vi "updatestats.vi"(8 "error in (no error)":errorcluster, 10 "Stats Ref":refnum<vi>, 11 "Result Ref":refnum<vi>) -> (0 "error IO":errorcluster, 3 "result ref out":refnum<vi>)   [LabVIEW 2022 SP3]
uses:
  <vilib>/Analysis/NI_AALBase.lvlib
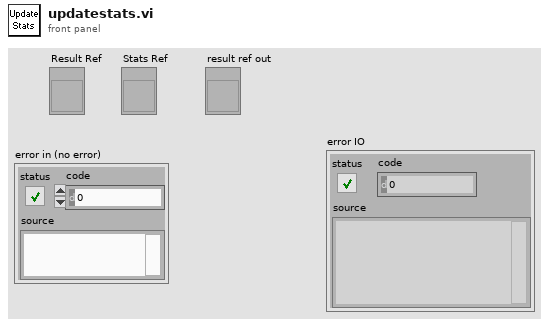
[diagram p1: front panel]
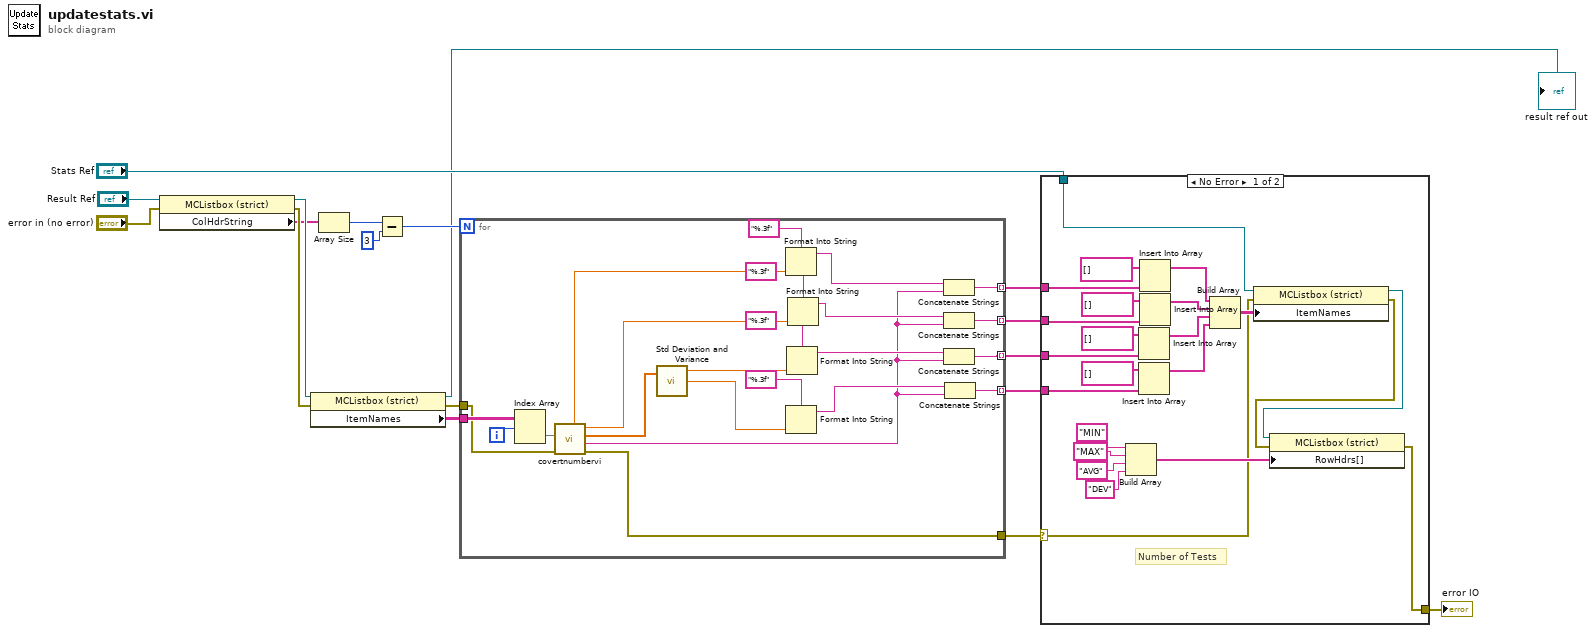
[diagram p0: block diagram]
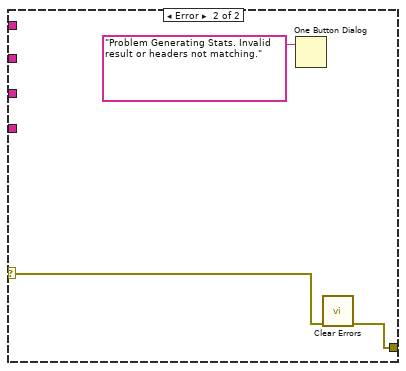
[diagram p2: hidden frame]
diagram:
  n1 = property class="MCListbox (strict)"(reference="Result Ref", error in="error in (no error)") -> (reference out=w15:refnum<vi>, error out=w18:errorcluster, "ColHdrString"=w14:string[])
  n2 = property class="MCListbox (strict)"(reference=w15, error in=w18) -> (reference out=→"result ref out":refnum<vi>, error out=w17:errorcluster, "ItemNames"=w16:string[][])
  n3 = Array Size(array=w14) -> (size(s)=w10:i32)
  n4 = Subtract(x=w10, y=u32 3) -> (x-y=w7:u32)
  n5 = for {
    N: w7 -> [_]
    tunnel: w16 -> [w41]
    tunnel: w17 -> [w28]
    tunnel: [w29] -> w13
    tunnel: [w32] -> w8 mode=indexing
    tunnel: [w31] -> w9 mode=indexing
    tunnel: [w37] -> w11 mode=indexing
    tunnel: [w34] -> w12 mode=indexing
    i -> [w40]
    n6 = Index Array(array=w41, index (col)=w40) -> (element=w27:string[])  [unwired: 1 in]
    n7 = call "covertnumbervi.vi"("error in"=w28, "Array"=w27) -> ("error out"=w29:errorcluster, "Symbol"=w26:string, "Array Out"=w23:dbl[], "max value"=w24:dbl, "min value"=w25:dbl)  [unwired: 4 in]
    n8 = call <vilib>:"Std Deviation and Variance.vi"("X"=w23) -> ("mean"=w38:dbl, "standard deviation"=w36:dbl)  [unwired: 1 in, 1 out]
    n9 = Format Into String(format string="%.3f", w25) -> (resulting string=w33:string)  [unwired: 2 in, 1 out]
    n10 = Format Into String(format string="%.3f", w36) -> (resulting string=w35:string)  [unwired: 2 in, 1 out]
    n11 = Format Into String(format string="%.3f", w38) -> (resulting string=w39:string)  [unwired: 2 in, 1 out]
    n12 = Format Into String(format string="%.3f", w24) -> (resulting string=w30:string)  [unwired: 2 in, 1 out]
    n13 = Concatenate Strings(w33, w26) -> (w32:string)
    n14 = Concatenate Strings(w30, w26) -> (w31:string)
    n15 = Concatenate Strings(w39, w26) -> (w37:string)
    n16 = Concatenate Strings(w35, w26) -> (w34:string)
  }
  n17 = case shown="No Error" w13 {
    selector: w13 -> [w45 w66]
    tunnel: [w47 w65] -> w2
    tunnel: w8 -> [w58 _]
    tunnel: w9 -> [w57 _]
    tunnel: w11 -> [w54 _]
    tunnel: w12 -> [w52 _]
    tunnel: "Stats Ref" -> [w50 _]
    frame No Error {
      # "Number of Tests"
      n18 = Build Array("MIN", "MAX", "AVG", "DEV") -> (w48:string[])
      n19 = Insert Into Array(array=string[] [], new element=w54) -> (w55:string[])  [unwired: 1 in]
      n20 = Insert Into Array(array=string[] [], new element=w52) -> (w51:string[])  [unwired: 1 in]
      n21 = Insert Into Array(array=string[] [], new element=w58) -> (w43:string[])  [unwired: 1 in]
      n22 = Insert Into Array(array=string[] [], new element=w57) -> (w42:string[])  [unwired: 1 in]
      n23 = Build Array(w43, w42, w55, w51) -> (w49:string[][])
      n24 = property class="MCListbox (strict)"(reference=w50, error in=w45, "ItemNames"=w49) -> (reference out=w44:refnum<vi>, error out=w46:errorcluster)
      n25 = property class="MCListbox (strict)"(reference=w44, error in=w46, "RowHdrs[]"=w48) -> (error out=w47:errorcluster)  [unwired: 1 out]
    }
    frame Error {
      n26 = One Button Dialog(message="Problem Generating Stats. Invalid result or headers not matching.") -> ()  [unwired: 1 in, 1 out]
      n27 = call <vilib>:"Clear Errors.vi"("error in (no error)"=w66) -> ("error out"=w65:errorcluster)  [unwired: 5 in, 1 out]
    }
  }
  "error IO" <- w2
